vi "EMV T6 Flow Detect.vi"(8 "error in (no error)":errorcluster, 10 "T6_DELTA_FLOW_THRESHOLD":dbl=4.0, 11 "T6 Temp":dbl=140.0) -> (0 "error out":errorcluster, 1 "Slope History":dbl[](array[numeric]), 2 "Flow Dectection":bool, 5 "Current T6 Temperatures Output":dbl[](array[numeric])=[75.0, 75.0, 75.0, 75.0, 75.0, 75.0, 75.0, 75.0, 75.0, 75.0, 75.0])   [LabVIEW 2016]
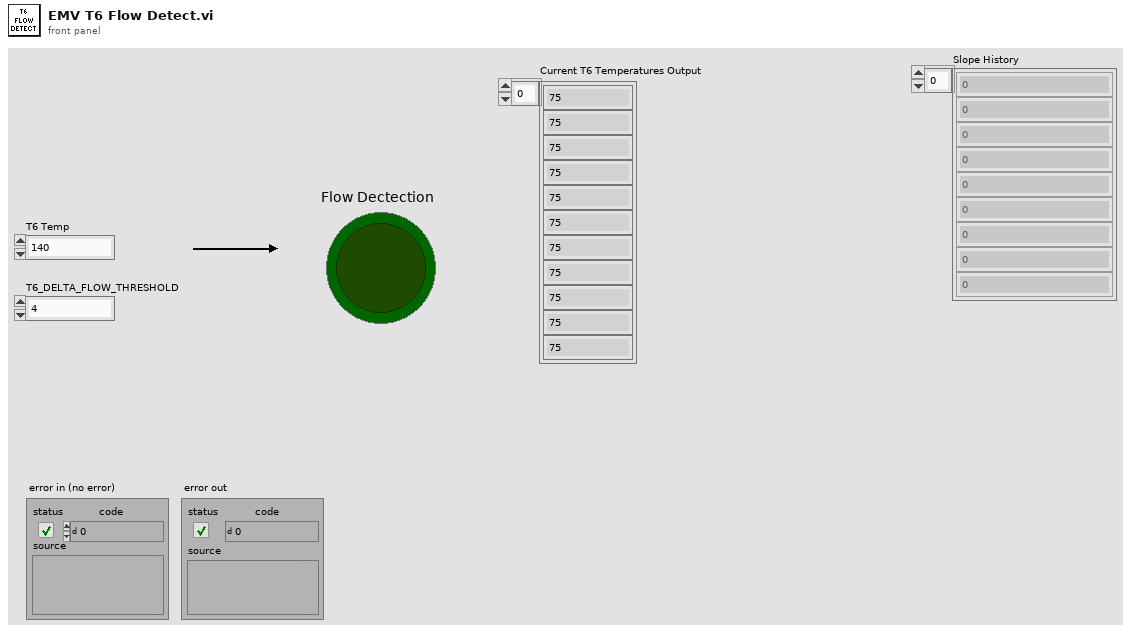
[diagram p1: front panel]
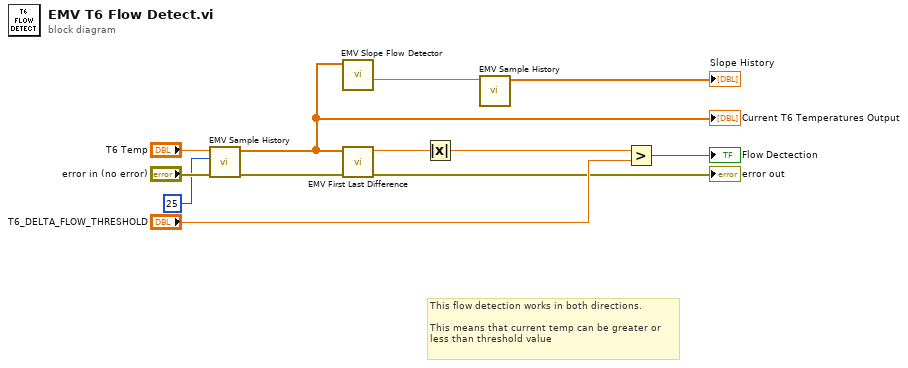
[diagram p0: block diagram]
diagram:
  # "This flow detection works in both directions.\n\nThis means that current temp can be greater or\nless than threshold value"
  n1 = call "EMV Sample History.vi"("error in (no error)"="error in (no error)", "length"=25, "T6 Temp"="T6 Temp") -> ("error out"=w5:errorcluster, "T6 History"=w7:dbl[])  [unwired: 7 in]
  "Current T6 Temperatures Output" <- w7
  n2 = call "EMV Slope Flow Detector.vi"("Current T6 Temperatures in"=w7) -> ("slope"=w3:dbl)  [unwired: 8 in, 2 out]
  n3 = call "EMV First Last Difference.vi"("error in (no error)"=w5, "Current T6 Temperatures in"=w7) -> ("error out"=→"error out":errorcluster, "First - Row 10"=w9:dbl)  [unwired: 5 in, 3 out]
  n4 = Absolute Value(x=w9) -> (abs(x)=w8:dbl)
  n5 = call "EMV Sample History.vi"("T6 Temp"=w3) -> ("T6 History"=→"Slope History":dbl[])  [unwired: 9 in, 1 out]
  n6 = Greater?(x=w8, y="T6_DELTA_FLOW_THRESHOLD") -> (0:→"Flow Dectection":bool)
